vi "Camera_IMAQdx_Create.vi"(8 "error in (no error)":errorcluster, 10 "Configuration":T1 {"Image Type" items=["Grayscale (U8)", "Grayscale (I16)", "Grayscale (SGL)", "Complex (CSG)", "RGB (U32)", "HSL (U32)", "RGB (U64)", "Grayscale (U16)"]}, 11 "reference in":refnum<class "Camera_IMAQdx.lvclass">) -> (0 "error out":errorcluster, 3 "reference out":refnum<class "Camera_IMAQdx.lvclass">)   [LabVIEW 2017, in "Camera_IMAQdx.lvclass"]
uses:
  Camera_IMAQdx.lvclass
  C:/VIT/simpleImageProcessingExample/lv_src/Camera/Camera_class/Camera.lvclass
  typedefs/Configuration--Cluster.ctl
  Camera_class/Camera.lvclass
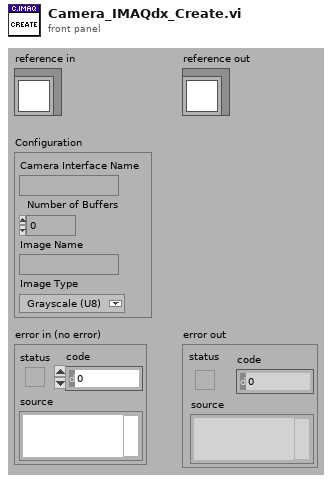
[diagram p1: front panel]
types:
  T1 = typedef "Camera_IMAQdx.lvclass/Configuration--Cluster.ctl" = cluster{"Camera Interface Name":string, "Number of Buffers":u32, "Image Name":string, "Image Type":T2}
  T2 = typedef "Image Type" = u32
  T3 = typedef "Camera_IMAQdx.lvclass/ObjectAttributes.ctl" = cluster{"Configuration":T1, "Session":T4, "Connected":bool, "Image":T5, "Frame Number":u32}
  T4 = typedef "IMAQdx.ctl" = refnum<k21>
  T5 = typedef "IMAQ Image.ctl" = refnum<image>
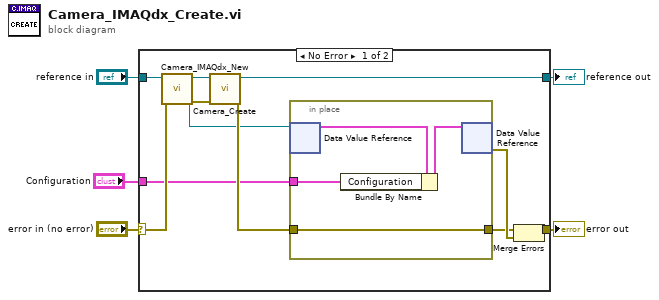
[diagram p0: block diagram]
diagram:
  n1 = case shown="No Error" "error in (no error)" {
    selector: "error in (no error)" -> [w10 w22]
    tunnel: [w12 w22] -> w4
    tunnel: "reference in" -> [w11 w21]
    tunnel: [w16 w21] -> w2
    tunnel: "Configuration" -> [w6 _]
    frame No Error {
      n2 = call "Camera_IMAQdx_New.vi"("error in (no error)"=w10, "reference in"=w11) -> ("error out"=w8:errorcluster, "DVRRefOut"=w7:refnum<data-value>, "reference out"=w9:refnum<class "Camera_IMAQdx.lvclass">)  [unwired: 6 in, 1 out]
      n3 = call "Camera_Create.vi"("error in (no error)"=w8, "reference in"=w9) -> ("error out"=w14:errorcluster, "reference out"=w16:refnum<class "Camera_IMAQdx.lvclass">)  [unwired: 8 in]
      n4 = in-place {
        in-place-border: w14 -> [w18]
        in-place-border: [w18] -> w13
        in-place-border: w6 -> [w17]
        n5 = in-place-dvr #1(w7) -> (w19:T3)  [unwired: 1 out]
        n6 = Bundle By Name(cluster=w19, "Configuration"=w17) -> (w20:T3)
        n7 = in-place-dvr #1(w20) -> (w15:errorcluster)  [unwired: 1 out]
      }
      n8 = Merge Errors(w13, w15) -> (w12:errorcluster)
    }
    frame Error {
      # "VI-TechBaseTemplate_Simple_4x4x4"
    }
  }
  "error out" <- w4
  "reference out" <- w2
